vi "Set Max Effort.vi"(8 "error in (no error)":errorcluster, 10 "max effort":dbl, 11 "Grips Robot in":refnum<class "Grips Robot.lvclass">) -> (0 "error out":errorcluster, 3 "Grips Robot out":refnum<class "Grips Robot.lvclass">)   [LabVIEW 2013, in "Grips Robot.lvclass"]
uses:
  Grips Robot.lvclass
  Grips Robot.lvclass/Grips Robot.ctl
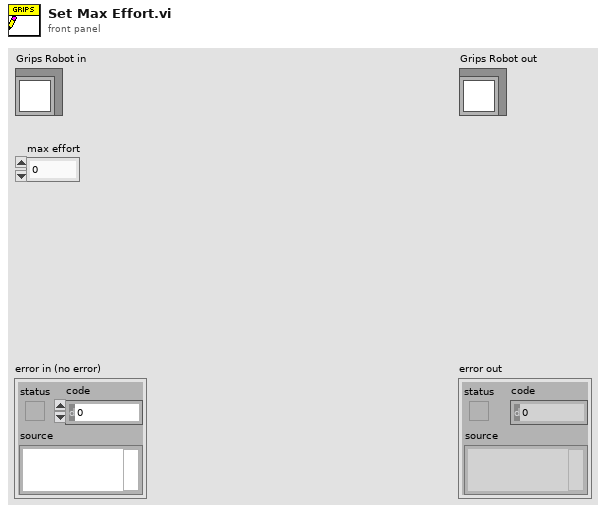
[diagram p1: front panel]
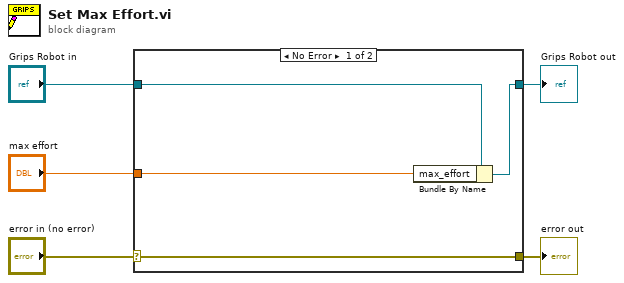
[diagram p0: block diagram]
diagram:
  n1 = case shown="No Error" "error in (no error)" {
    selector: "error in (no error)" -> [w9 w10]
    tunnel: [w9 w10] -> w4
    tunnel: [w7 w11] -> w2
    tunnel: "Grips Robot in" -> [w8 w11]
    tunnel: "max effort" -> [w6 _]
    frame No Error {
      n2 = Bundle By Name(cluster=w8, "max_effort"=w6) -> (w7:refnum<class "Grips Robot.lvclass">)
    }
    frame Error {
    }
  }
  "error out" <- w4
  "Grips Robot out" <- w2
